vi "Decode Enable.vi"(8 "error in (no error)":errorcluster) -> (0 "error out":errorcluster)   [LabVIEW 2019]
uses:
  Globals.vi
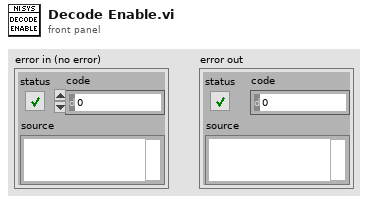
[diagram p1: front panel]
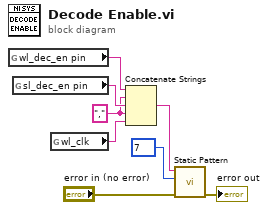
[diagram p0: block diagram]
diagram:
  w1 = "," ("string")
  n1 = global read "Globals.vi" "wl_dec_en pin"() -> (w4:string)
  n2 = global read "Globals.vi" "sl_dec_en pin"() -> (w3:string)
  n3 = global read "Globals.vi" "wl_clk"() -> (w2:string)
  n4 = Concatenate Strings(w4, w1, w3, w1, w2) -> (w5:string)
  n5 = call "Static Pattern.vi"("error in (no error)"="error in (no error)", "write data (0x0000)"=u32 7, "channel list (all:\"\")"=w5) -> ("error out"=→"error out":errorcluster)  [unwired: 8 in]
